vi "Parse NT Numeric Array.vi"(11 "TCP Network Connection in":refnum<k5>) -> (0 "String":string, 1 "Size":i32=1, 2 "Numeric Array":dbl[](array[numeric]), 3 "TCP Network Connection out":refnum<k5>)   [LabVIEW 2017]
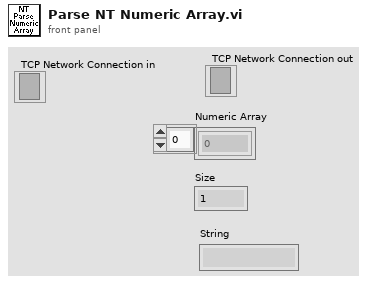
[diagram p1: front panel]
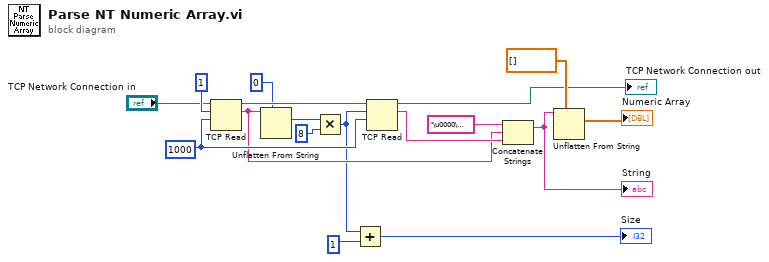
[diagram p0: block diagram]
diagram:
  w9 = 1000 ("timeout ms (25000)")
  n1 = TCP Read(connection ID="TCP Network Connection in", bytes to read=1 ("timeout ms (25000)"), 9:w9) -> (connection ID out=w12:refnum<k5>, data out=w5:string)  [unwired: 2 in, 1 out]
  n2 = Unflatten From String(type=u8 0 ("Size"), binary string=w5) -> (value=w7:u8)  [unwired: 3 in, 2 out]
  n3 = Multiply(x=w7, y=8 ("timeout ms (25000)")) -> (x*y=w1:i32)
  n4 = Add(x=w1, y=1 ("timeout ms (25000)")) -> (x+y=→"Size":i32)
  n5 = TCP Read(connection ID=w12, bytes to read=w1, 9:w9) -> (connection ID out=→"TCP Network Connection out":refnum<k5>, data out=w6:string)  [unwired: 2 in, 1 out]
  n6 = Concatenate Strings("\u0000\u0000\u0000", w5, w6) -> (w4:string)
  "String" <- w4
  n7 = Unflatten From String(type=dbl[] [], binary string=w4) -> (value=→"Numeric Array":dbl[])  [unwired: 3 in, 2 out]
